vi "Math SubVI - Medium (SCR).vi"(1 "Input":dbl step=0.1 format="%.6f") -> (0 "Output":dbl format="%.6f")   [LabVIEW 2026]
doc: "This VI takes a floating-point number between 0 and 1 and maps it to another floating-point number between 0 and 1."
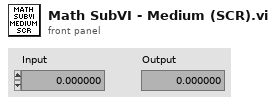
[diagram p1: front panel]
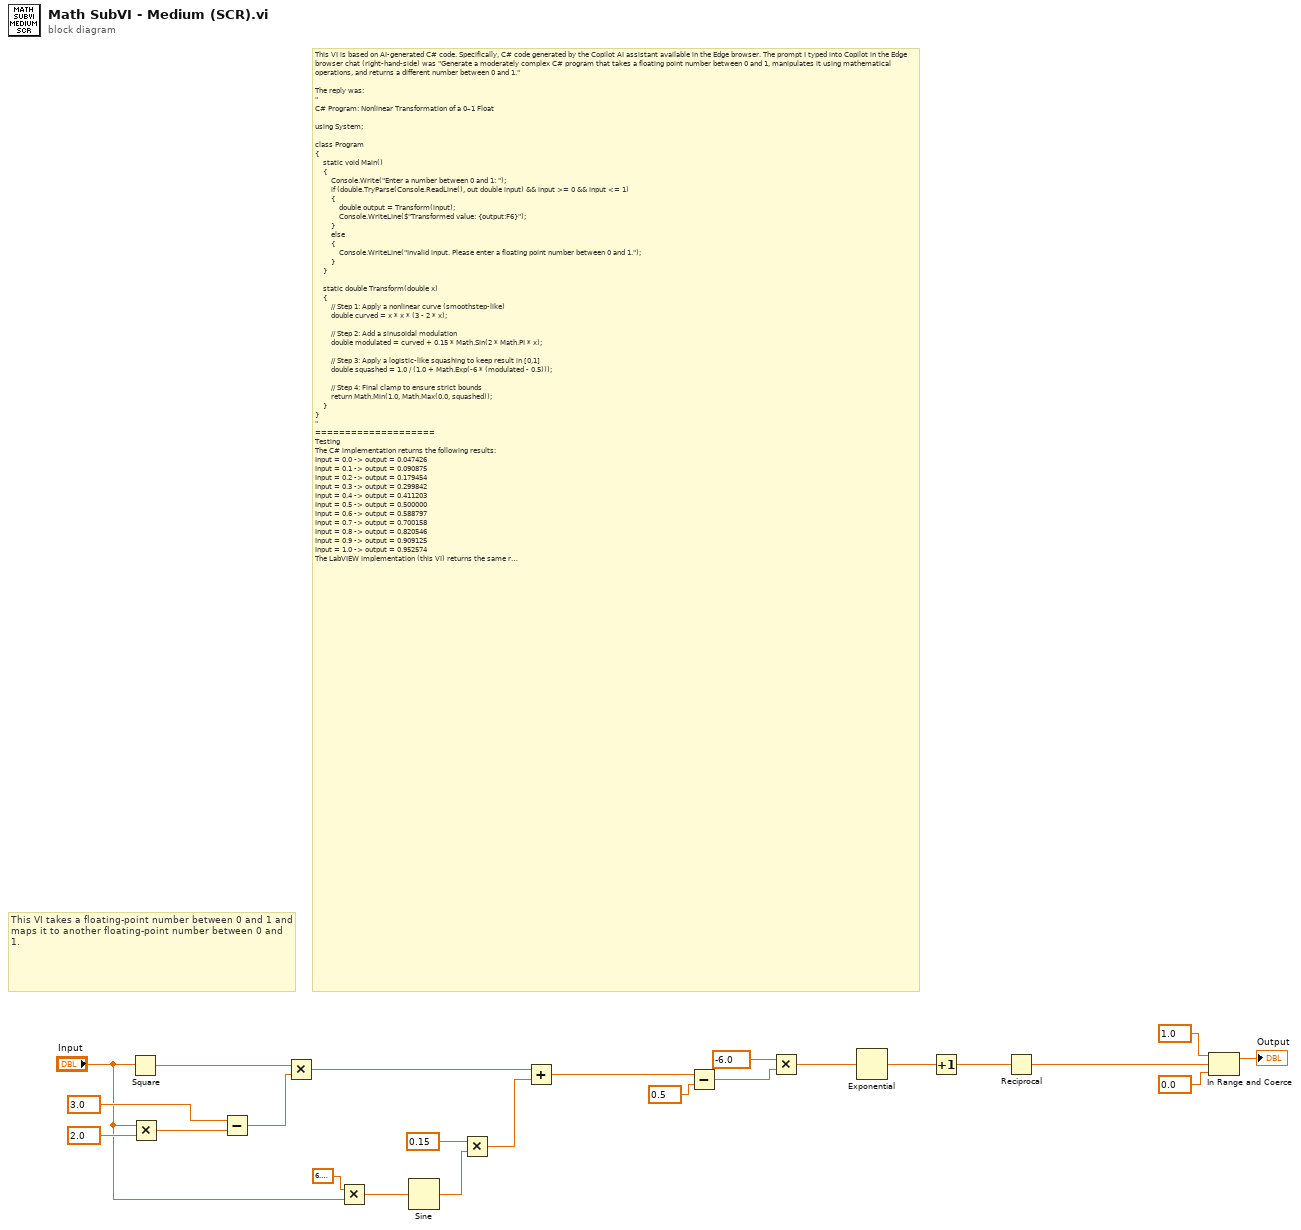
[diagram p0: block diagram]
diagram:
  # "This VI is based on AI-generated C# code. Specifically, C# code generated by the Copilot AI assistant available in the Edge browser. The prompt I typed into Copilot in the Edge browser chat (right-hand-side) was \"Generate a moderately complex C# program that takes a floating point number between 0 and 1, manipulates it using mathematical operations, and returns a different number between 0 and 1.\"\n\nThe reply was:\n\"\nC# Program: Nonlinear Transformation of a 0–1 Float\n\nusing System;\n\nclass Program\n{\n    static void Main()\n    {\n        Console.Write(\"Enter a number between 0 and 1: \");\n        if (double.TryParse(Console.ReadLine(), out double input) && input >= 0 && input <= 1)\n        {\n            double output = Transform(input);\n            Console.WriteLine($\"Transformed value: {output:F6}\");\n        }\n        else\n        {\n            Console.WriteLine(\"Invalid input. Please enter a floating point number between 0 and 1.\");\n        }\n    }\n\n    static double Transform(double x)\n    {\n        // Step 1: Apply a nonlinear curve (smoothstep-like)\n        double curved = x * x * (3 - 2 * x);\n\n        // Step 2: Add a sinusoidal modulation\n        double modulated = curved + 0.15 * Math.Sin(2 * Math.PI * x);\n\n        // Step 3: Apply a logistic-like squashing to keep result in [0,1]\n        double squashed = 1.0 / (1.0 + Math.Exp(-6 * (modulated - 0.5)));\n\n        // Step 4: Final clamp to ensure strict bounds\n        return Math.Min(1.0, Math.Max(0.0, squashed));\n    }\n}\n\"\n====================\nTesting\nThe C# implementation returns the following results:\nInput = 0.0 -> output = 0.047426\nInput = 0.1 -> output = 0.090875\nInput = 0.2 -> output = 0.179454\nInput = 0.3 -> output = 0.299842\nInput = 0.4 -> output = 0.411203\nInput = 0.5 -> output = 0.500000\nInput = 0.6 -> output = 0.588797\nInput = 0.7 -> output = 0.700158\nInput = 0.8 -> output = 0.820546\nInput = 0.9 -> output = 0.909125\nInput = 1.0 -> output = 0.952574\nThe LabVIEW implementation (this VI) returns the same results for the given inputs. This confirms that this VI is faithful to the C# code generated by Copilot.\n====================\nThis note last updated by: Petru Tarabuta, 06 September 2026"
  # "This VI takes a floating-point number between 0 and 1 and maps it to another floating-point number between 0 and 1."
  n1 = Square(x="Input") -> (x^2=w23:dbl)
  n2 = Multiply(x="Input", y=2.0 ("x")) -> (x*y=w20:dbl)
  n3 = Subtract(x=3.0, y=w20) -> (x-y=w19:dbl)
  n4 = Multiply(x=w23, y=w19) -> (x*y=w18:dbl)
  n5 = Multiply(x=6.283185307179586, y="Input") -> (x*y=w14:dbl)
  n6 = Sine(x=w14) -> (sin(x)=w13:dbl)
  n7 = Multiply(x=0.15, y=w13) -> (x*y=w12:dbl)
  n8 = Add(x=w18, y=w12) -> (x+y=w10:dbl)
  n9 = Subtract(x=w10, y=0.5 ("x")) -> (x-y=w9:dbl)
  n10 = Multiply(x=-6.0, y=w9) -> (x*y=w7:dbl)
  n11 = Exponential(1:w7) -> (0:w6:dbl)
  n12 = Increment(x=w6) -> (x+1=w5:dbl)
  n13 = Reciprocal(x=w5) -> (1/x=w4:dbl)
  n14 = In Range and Coerce(upper limit=1.0 ("x"), x=w4, lower limit=0.0 ("x")) -> (coerced(x)=→"Output":dbl)  [unwired: 1 out]
